vi "Untitled 2.vi"   [LabVIEW 2015]
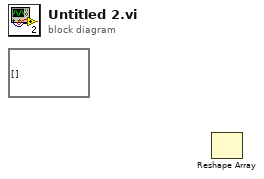
[diagram p0: block diagram]
diagram:
  (unwired) void[] []
  n1 = Reshape Array() -> ()  [unwired: 2 in, 1 out]
